vi "Status Count.vi"(0 "Status":i32[](array[numeric])) -> (1 "Dead":i32, 2 "Helathy":i32, 3 "Infected":i32)   [LabVIEW 2014]
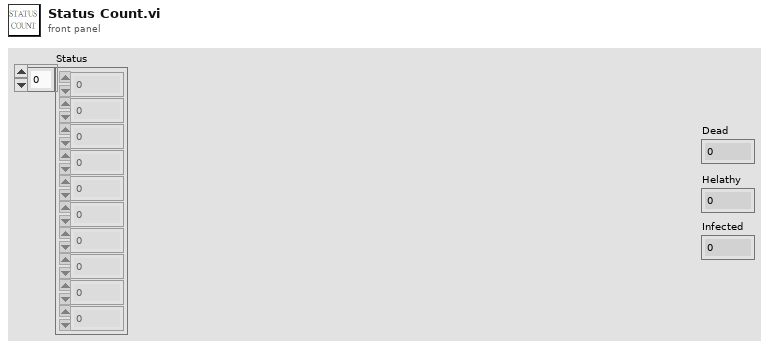
[diagram p1: front panel]
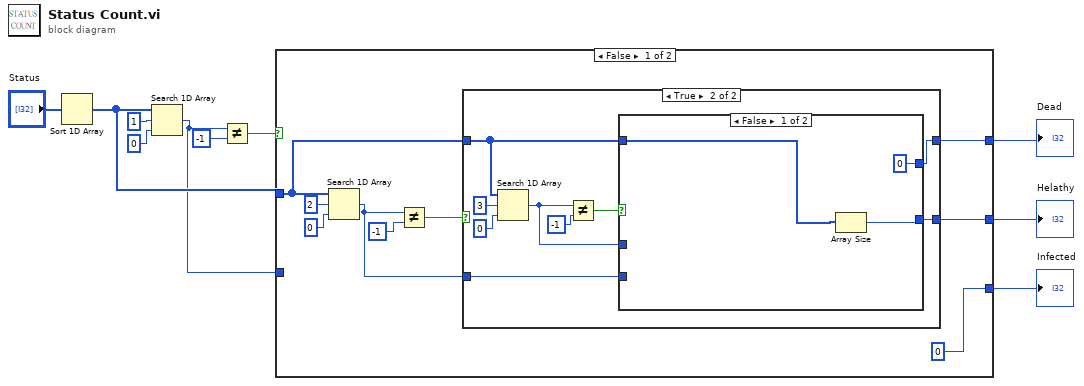
[diagram p0: block diagram]
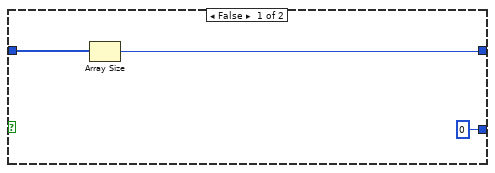
[diagram p2: hidden frame]
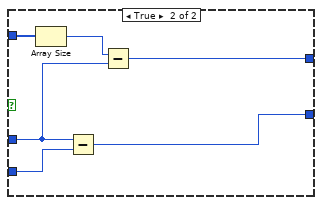
[diagram p3: hidden frame]
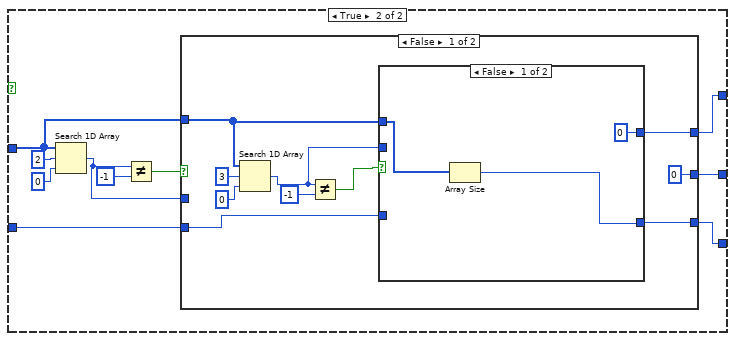
[diagram p4: hidden frame]
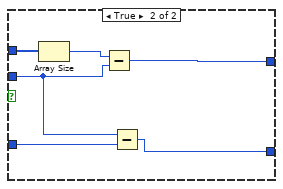
[diagram p5: hidden frame]
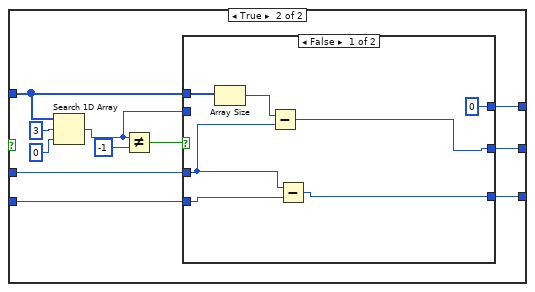
[diagram p6: hidden frame]
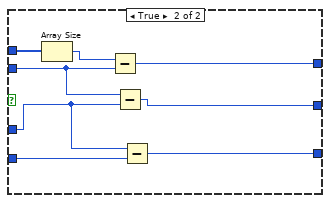
[diagram p7: hidden frame]
diagram:
  n1 = Sort 1D Array(array="Status") -> (sorted array=w5:i32[])
  n2 = Search 1D Array(1D array=w5, element=1, start index (0)=0) -> (index of element=w1:i32)
  n3 = Not Equal?(x=w1, y=-1) -> (x != y?=w6:bool)
  n4 = case shown="False" w6 {
    tunnel: w5 -> [w15 w46]
    tunnel: [w14 w41] -> w4
    tunnel: [w12 w42] -> w3
    tunnel: [0 w43] -> w2
    tunnel: w1 -> [_ w44]
    frame False {
      n5 = Search 1D Array(1D array=w15, element=2, start index (0)=0) -> (index of element=w13:i32)
      n6 = Not Equal?(x=w13, y=-1) -> (x != y?=w16:bool)
      n7 = case shown="True" w16 {
        tunnel: w15 -> [w22 w24]
        tunnel: [w21 w23] -> w14
        tunnel: w13 -> [_ w26]
        tunnel: [0 w25] -> w12
        frame False {
          n8 = Array Size(array=w22) -> (size(s)=w21:i32)
        }
        frame True {
          n9 = Search 1D Array(1D array=w24, element=3, start index (0)=0) -> (index of element=w27:i32)
          n10 = Not Equal?(x=w27, y=-1) -> (x != y?=w28:bool)
          n11 = case shown="False" w28 {
            tunnel: w27 -> [_ w36]
            tunnel: w26 -> [_ w40]
            tunnel: [w33 w39] -> w25
            tunnel: w24 -> [w32 w38]
            tunnel: [0 w35] -> w23
            frame False {
              n12 = Array Size(array=w32) -> (size(s)=w33:i32)
            }
            frame True {
              n13 = Array Size(array=w38) -> (size(s)=w37:i32)
              n14 = Subtract(x=w36, y=w40) -> (x-y=w39:i32)
              n15 = Subtract(x=w37, y=w36) -> (x-y=w35:i32)
            }
          }
        }
      }
    }
    frame True {
      n16 = Search 1D Array(1D array=w46, element=2, start index (0)=0) -> (index of element=w45:i32)
      n17 = Not Equal?(x=w45, y=-1) -> (x != y?=w47:bool)
      n18 = case shown="False" w47 {
        tunnel: w46 -> [w55 w76]
        tunnel: w45 -> [_ w74]
        tunnel: w44 -> [w52 w73]
        tunnel: [w51 w72] -> w43
        tunnel: [0 w71] -> w42
        tunnel: [w53 w70] -> w41
        frame False {
          n19 = Search 1D Array(1D array=w55, element=3, start index (0)=0) -> (index of element=w54:i32)
          n20 = Not Equal?(x=w54, y=-1) -> (x != y?=w57:bool)
          n21 = case shown="False" w57 {
            tunnel: w55 -> [w62 w69]
            tunnel: w54 -> [_ w66]
            tunnel: [0 w67] -> w53
            tunnel: w52 -> [_ w65]
            tunnel: [w61 w64] -> w51
            frame False {
              n22 = Array Size(array=w62) -> (size(s)=w61:i32)
            }
            frame True {
              n23 = Array Size(array=w69) -> (size(s)=w68:i32)
              n24 = Subtract(x=w68, y=w66) -> (x-y=w67:i32)
              n25 = Subtract(x=w66, y=w65) -> (x-y=w64:i32)
            }
          }
        }
        frame True {
          n26 = Search 1D Array(1D array=w76, element=3, start index (0)=0) -> (index of element=w75:i32)
          n27 = Not Equal?(x=w75, y=-1) -> (x != y?=w77:bool)
          n28 = case shown="False" w77 {
            tunnel: w76 -> [w86 w95]
            tunnel: w75 -> [_ w93]
            tunnel: w74 -> [w83 w91]
            tunnel: w73 -> [w82 w92]
            tunnel: [w81 w90] -> w72
            tunnel: [w84 w89] -> w71
            tunnel: [0 w88] -> w70
            frame False {
              n29 = Array Size(array=w86) -> (size(s)=w85:i32)
              n30 = Subtract(x=w85, y=w83) -> (x-y=w84:i32)
              n31 = Subtract(x=w83, y=w82) -> (x-y=w81:i32)
            }
            frame True {
              n32 = Array Size(array=w95) -> (size(s)=w94:i32)
              n33 = Subtract(x=w94, y=w93) -> (x-y=w88:i32)
              n34 = Subtract(x=w93, y=w91) -> (x-y=w89:i32)
              n35 = Subtract(x=w91, y=w92) -> (x-y=w90:i32)
            }
          }
        }
      }
    }
  }
  "Dead" <- w4
  "Helathy" <- w3
  "Infected" <- w2
